vi "LHF.DB.Mongo.Util.HandleJSONTextTag.vi"(11 "Variant Data":T1) -> (2 "tagged as JSON text":bool, 3 "Variant Data (tag stripped)":T1)   [LabVIEW 2013, in "LHF.DB.Mongo.lvclass"]
uses:
  LHF.DB.Mongo.lvclass
  Typedef/LHF.DB.Mongo.Typedef.VariantData.ctl
  <vilib>/Utility/VariantDataType/Type.ctl
  <vilib>/Utility/VariantDataType/VariantType.lvlib
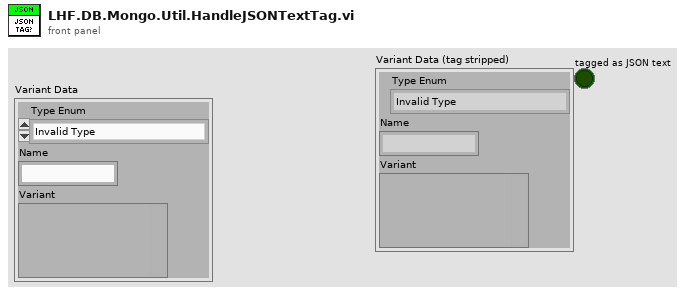
[diagram p1: front panel]
types:
  T1 = typedef "LHF.DB.Mongo.lvclass/LHF.DB.Mongo.Typedef.VariantData.ctl" = cluster{"Type Enum":T2, "Name":string, "Variant":variant}
  T2 = typedef "VariantType.lvlib/Type.ctl" = enum8{"Invalid Type", "Void", "I8", "I16", "I32", "I64", "U8", "U16", "U32", "U64", "Single Float", "Double Float", "Extended Float", "Single Complex", "Double Complex", "Extended Complex", "Enum U8", "Enum U16", "Enum U32", "Enum U64", "Single Float With Unit", "Double Float With Unit", "Extended Float With Unit", "Single Complex with Unit", "Double Complex with Unit", "Extended Complex with Unit", "Boolean", "String", "Path", "Picture", "Tag", "Array", "Cluster", "Variant", "LV Variant", "Waveform", "Timestamp", "Digital Waveform", "Digital Data", "ExpressData", "Refnum", "External Data", "VI", "Poly VI", "LabVIEW Class Instance", "Fixed Point"}
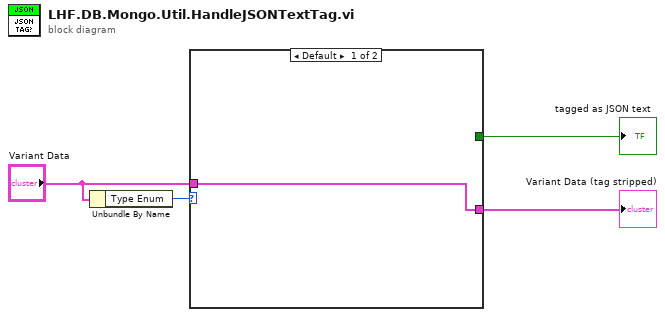
[diagram p0: block diagram]
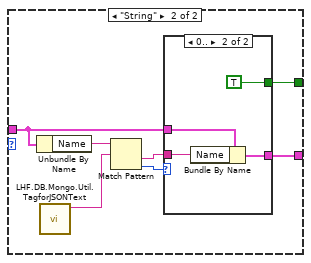
[diagram p2: hidden frame]
diagram:
  n1 = Unbundle By Name("Variant Data") -> ("Type Enum"=w4:T2)
  n2 = case shown="Default" w4 {
    tunnel: [w5 w11] -> w2
    tunnel: "Variant Data" -> [w5 w9]
    tunnel: [_ w7] -> w1
    frame Default {
    }
    frame "String" {
      n3 = Unbundle By Name(w9) -> ("Name"=w8:string)
      n4 = call "LHF.DB.Mongo.Util.TagforJSONText.vi"() -> ("Tag for JSON text"=w6:string)  [unwired: 11 in]
      n5 = Match Pattern(string=w8, regular expression=w6) -> (after substring=w10:string, offset past match=w12:i32)  [unwired: 1 in, 2 out]
      n6 = case shown="0.." w12 {
        tunnel: [w13 w16] -> w11
        tunnel: w9 -> [w13 w17]
        tunnel: w10 -> [_ w15]
        tunnel: [_ TRUE] -> w7
        frame ..-1 {
        }
        frame 0.. {
          n7 = Bundle By Name(cluster=w17, "Name"=w15) -> (w16:T1)
        }
      }
    }
  }
  "Variant Data (tag stripped)" <- w2
  "tagged as JSON text" <- w1
